vi "lee_ee.vi"(0 "Volt?":enum32{"492", "1492", "307", "568"}(ring), 4 "EE 568 S IN":T1(array[cluster]) {"Analogicas 32"."?" items=["1", "2", "4", "8", "16", "32", "64", "128", "256"]; "Analogicas 32"."?" items=["Lineal"=15, "Cuadrática"=14]; "Analogicas 32"."unsigned byte array[0]" items=["10000", "1000", "100", "10", "8000", "800", "80", "8", "4000", "400", "40", "4", "2000", "200", "20", "2"]; "Analogicas 16"."?" items=["1", "2", "4", "8", "16", "32", "64", "128", "256"]; "Analogicas 16"."?" items=["Lineal"=15, "Cuadrática"=14]; "Analogicas 16"."unsigned byte array[0]" items=["10000", "1000", "100", "10", "8000", "800", "80", "8", "4000", "400", "40", "4", "2000", "200", "20", "2"]}, 5 "Exe path":string, 6 "Nº equipo":i32, 7 "Config Equipos":T2(array[cluster]) {"Ref PD 2" max=10000 step=1; "Med Princ" items=["1", "2", "3", "4", "5", "6", "7", "8", "9", "10", "11", "12", "13", "14", "15", "16", "17", "18", "19", "20", "21", "22", "23", "24", "25", "26", "27", "28", "29", "30", "31", "32"]}, 8 "EE 492 IN":T3(array[cluster]), 9 "EE 568 M IN":T1(array[cluster]) {"Analogicas 32"."?" items=["1", "2", "4", "8", "16", "32", "64", "128", "256"]; "Analogicas 32"."?" items=["Lineal"=15, "Cuadrática"=14]; "Analogicas 32"."unsigned byte array[0]" items=["10000", "1000", "100", "10", "8000", "800", "80", "8", "4000", "400", "40", "4", "2000", "200", "20", "2"]; "Analogicas 16"."?" items=["1", "2", "4", "8", "16", "32", "64", "128", "256"]; "Analogicas 16"."?" items=["Lineal"=15, "Cuadrática"=14]; "Analogicas 16"."unsigned byte array[0]" items=["10000", "1000", "100", "10", "8000", "800", "80", "8", "4000", "400", "40", "4", "2000", "200", "20", "2"]}) -> (1 "EE 568 S OUT":T1(array[cluster]) {"Analogicas 32"."?" items=["1", "2", "4", "8", "16", "32", "64", "128", "256"]; "Analogicas 32"."?" items=["Lineal"=15, "Cuadrática"=14]; "Analogicas 32"."unsigned byte array[0]" items=["10000", "1000", "100", "10", "8000", "800", "80", "8", "4000", "400", "40", "4", "2000", "200", "20", "2"]; "Analogicas 16"."?" items=["1", "2", "4", "8", "16", "32", "64", "128", "256"]; "Analogicas 16"."?" items=["Lineal"=15, "Cuadrática"=14]; "Analogicas 16"."unsigned byte array[0]" items=["10000", "1000", "100", "10", "8000", "800", "80", "8", "4000", "400", "40", "4", "2000", "200", "20", "2"]}, 2 "EE 492 OUT":T3(array[cluster]), 3 "EE 568 M OUT":T1(array[cluster]) {"Analogicas 32"."?" items=["1", "2", "4", "8", "16", "32", "64", "128", "256"]; "Analogicas 32"."?" items=["Lineal"=15, "Cuadrática"=14]; "Analogicas 32"."unsigned byte array[0]" items=["10000", "1000", "100", "10", "8000", "800", "80", "8", "4000", "400", "40", "4", "2000", "200", "20", "2"]; "Analogicas 16"."?" items=["1", "2", "4", "8", "16", "32", "64", "128", "256"]; "Analogicas 16"."?" items=["Lineal"=15, "Cuadrática"=14]; "Analogicas 16"."unsigned byte array[0]" items=["10000", "1000", "100", "10", "8000", "800", "80", "8", "4000", "400", "40", "4", "2000", "200", "20", "2"]})   [LabVIEW 2010]
panel:
  out "err":errorcluster
  out "error out":errorcluster
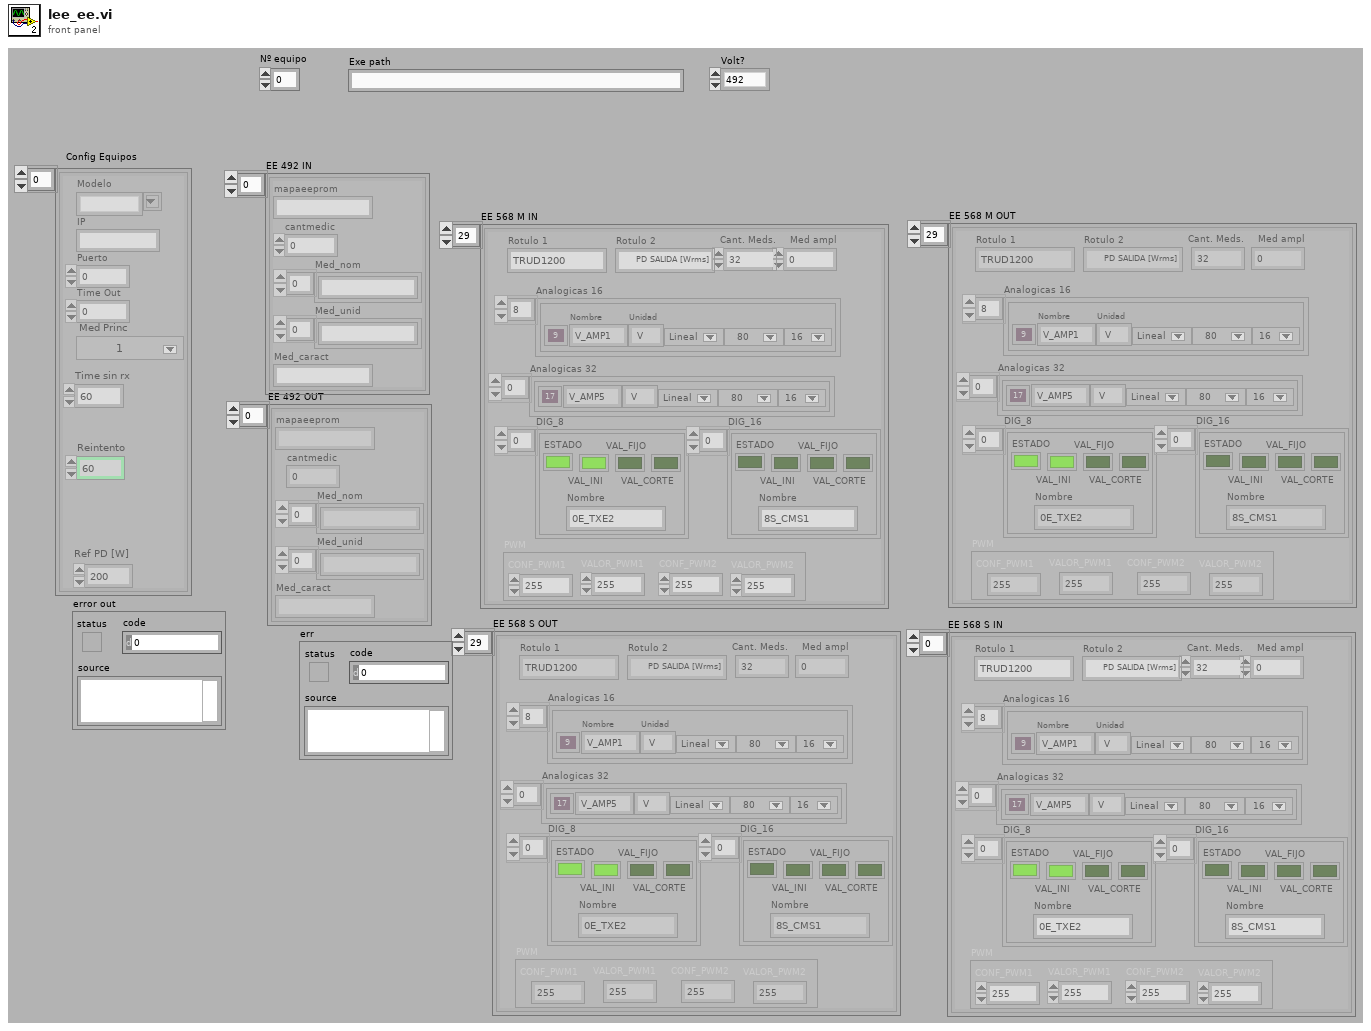
[diagram p1: front panel]
types:
  T1 = cluster{"Rotulo 1":string, "Rotulo 2":string, "Cant. Meds.":u8, "Med ampl":u8, "Analogicas 16":cluster{"Nº":i32, "Nombre":string, "Unidad":string, u8, "unsigned byte array[0]":u8, u8}[], "Analogicas 32":cluster{i32, "mapaeeprom":string, "mapaeeprom":string, u8, "unsigned byte array[0]":u8, u8}[], "DIG_8":cluster{"ESTADO":bool, "VAL_INI":bool, "VAL_FIJO":bool, "VAL_CORTE":bool, "Nombre":string}[], "DIG_16":cluster{"ESTADO":bool, "VAL_INI":bool, "VAL_FIJO":bool, "VAL_CORTE":bool, "Nombre":string}[], "PWM":cluster{"CONF_PWM1":u8, "VALOR_PWM1":u8, "CONF_PWM2":u8, "VALOR_PWM2":u8}}[]
  T2 = cluster{"Modelo":string, "IP":string, "Puerto":u16, "Time Out":u16, "Med Princ":u16, "Time sin rx":u16, "Reintento":u16, "Ref PD 2":u16}[]
  T3 = cluster{"mapaeeprom":string, "cantmedic":u8, "Med_nom":string[], "Med_unid":string[], "Med_caract":string}[]
  T4 = cluster{"Modelo":string, "IP":string, "Puerto":u16, "Time Out":u16, "Med Princ":u16, "Time sin rx":u16, "Reintento":u16, "Ref PD 2":u16}
  T5 = cluster{string, "cantmedic":u8, "Med_nom":string[], "Med_unid":string[], "Med_caract":string}
  T6 = cluster{"Rotulo 1":string, "Rotulo 2":string, "Cant. Meds.":u8, "Med ampl":u8, "Analogicas 16":cluster{i32, "mapaeeprom":string, "mapaeeprom":string, u8, "unsigned byte array[0]":u8, u8}[], "Analogicas 32":cluster{i32, "mapaeeprom":string, "mapaeeprom":string, u8, "unsigned byte array[0]":u8, u8}[], "DIG_CARACT":cluster{"ESTADO":bool, "VAL_INI":bool, "VAL_FIJO":bool, "VAL_CORTE":bool, "CARACT LOG 9-16":string}[], "DIG_CARACT 2":cluster{"ESTADO":bool, "VAL_INI":bool, "VAL_FIJO":bool, "VAL_CORTE":bool, "CARACT LOG 9-16":string}[], "PWM":cluster{"CONF_PWM1":u8, "VALOR_PWM1":u8, "CONF_PWM2":u8, "VALOR_PWM2":u8}}
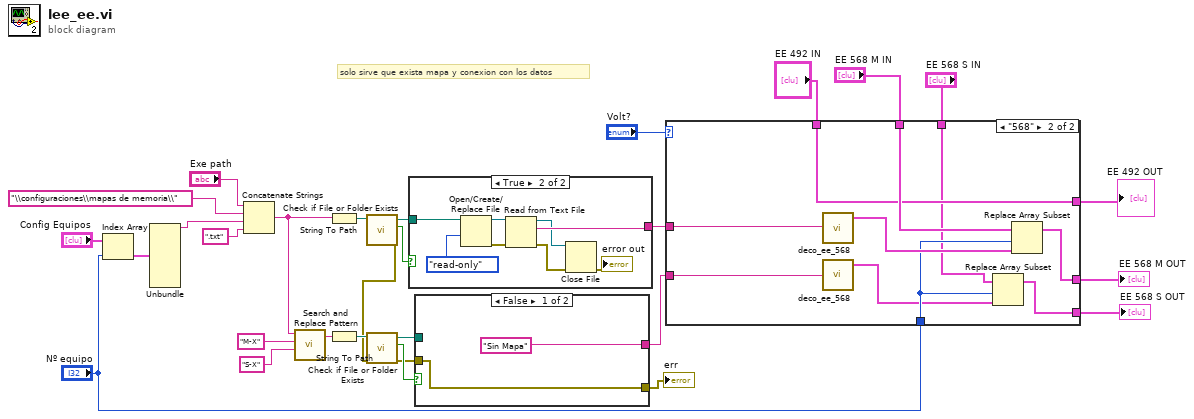
[diagram p0: block diagram]
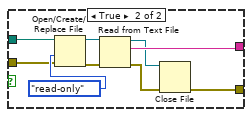
[diagram p2: hidden frame]
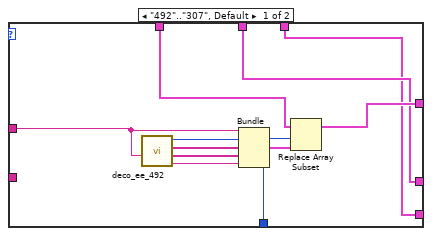
[diagram p3: hidden frame]
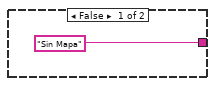
[diagram p4: hidden frame]
diagram:
  # "solo sirve que exista mapa y conexion con los datos"
  n1 = Index Array(array="Config Equipos", index="Nº equipo") -> (element=w22:T4)
  n2 = Unbundle(w22) -> ("Modelo"=w19:string)  [unwired: 7 out]
  n3 = Concatenate Strings("Exe path", "\\configuraciones\\mapas de memoria\\" ("replace string (\"\")"), w19, ".txt" ("string")) -> (w11:string)
  n4 = call <vilib>:"Search and Replace Pattern.vi"("string"=w11, "regular expression (\"\")"="M-X" ("regular expression (\"\")"), "replace string (\"\")"="S-X" ("regular expression (\"\")")) -> ("result string"=w6:string)  [unwired: 2 in, 1 out]
  n5 = String To Path(string=w11) -> (path=w24:path)
  n6 = String To Path(string=w6) -> (path=w9:path)
  n7 = call <vilib>:"Check if File or Folder Exists.vi"("path"=w24) -> ("error out"=w4:errorcluster, "file or folder exists?"=w23:bool, "dup path"=w28:path)  [unwired: 1 in, 7 out]
  n8 = call <vilib>:"Check if File or Folder Exists.vi"("error in (no error)"=w4, "path"=w9) -> ("error out"=w3:errorcluster, "file or folder exists?"=w10:bool, "dup path"=w8:path)  [unwired: 7 out]
  n9 = case shown="True" w23 {
    tunnel: w28 -> [_ w38]
    tunnel: ["Sin Mapa" w35] -> w29
    frame False {
    }
    frame True {
      n10 = Open/Create/Replace File(file path (use dialog)=w38, access (0:read/write)=enum16{"read/write", "read-only", "write-only"}."read-only") -> (refnum out=w37:refnum<file>, error out=w36:errorcluster)  [unwired: 2 in, 3 out]
      n11 = Read from Text File(file (use dialog)=w37, error in=w36) -> (refnum out=w34:refnum<file>, text=w35:string, error out=w33:errorcluster)  [unwired: 3 out]
      n12 = Close File(refnum=w34, error in=w33) -> (error out=→"error out":errorcluster)  [unwired: 1 out]
    }
  }
  n13 = case shown="False" w10 {
    tunnel: w8 -> [_ w49]
    tunnel: ["Sin Mapa" w46] -> w7
    tunnel: w3 -> [w39 w42]
    tunnel: [w39 w41] -> w2
    frame False {
    }
    frame True {
      n14 = Open/Create/Replace File(file path (use dialog)=w49, error in=w42, access (0:read/write)=enum16{"read/write", "read-only", "write-only"}."read-only") -> (refnum out=w48:refnum<file>, error out=w47:errorcluster)  [unwired: 1 in, 3 out]
      n15 = Read from Text File(file (use dialog)=w48, error in=w47) -> (refnum out=w45:refnum<file>, text=w46:string, error out=w44:errorcluster)  [unwired: 3 out]
      n16 = Close File(refnum=w45, error in=w44) -> (error out=w41:errorcluster)  [unwired: 1 out]
    }
  }
  "err" <- w2
  n17 = case shown="\"568\"" "Volt?" {
    tunnel: w29 -> [w55 w63]
    tunnel: "Nº equipo" -> [w54 w65]
    tunnel: "EE 492 IN" -> [w53 w67]
    tunnel: [w52 w67] -> w17
    tunnel: "EE 568 M IN" -> [w51 w69]
    tunnel: [w51 w68] -> w15
    tunnel: [w50 w66] -> w14
    tunnel: w7 -> [_ w62]
    tunnel: "EE 568 S IN" -> [w50 w61]
    frame "492".."307", Default {
      n18 = call "deco_ee_492.vi"("mapaeeprom"=w55) -> ("Med_caract"=w59:string, "Med_unid"=w58:string[], "Med_nom"=w57:string[], "cantmedic"=w56:u8)  [unwired: 3 in]
      n19 = Bundle(w55, "cantmedic"=w56, "Med_nom"=w57, "Med_unid"=w58, "Med_caract"=w59) -> (w60:T5)  [unwired: 1 out]
      n20 = Replace Array Subset(array=w53, new element=w60, index=w54) -> (w52:T3)
    }
    frame "568" {
      n21 = call "deco_ee_568.vi"("data IN"=w63) -> ("Eeprom"=w70:T6)  [unwired: 2 in, 2 out]
      n22 = call "deco_ee_568.vi"("data IN"=w62) -> ("Eeprom"=w64:T6)  [unwired: 2 in, 2 out]
      n23 = Replace Array Subset(array=w61, new element=w64, index=w65) -> (w66:T1)
      n24 = Replace Array Subset(array=w69, new element=w70, index=w65) -> (w68:T1)
    }
  }
  "EE 492 OUT" <- w17
  "EE 568 M OUT" <- w15
  "EE 568 S OUT" <- w14
